vi "GetHeuristicCost.vi"(8 "error in (no error)":errorcluster, 10 "Goal NodeReference":refnum<data-value>, 11 "AbstractAstarNode in":refnum<class "NI_Robotics_AbstractAstarNode.lvclass">) -> (0 "error out":errorcluster, 2 "hueristic cost":dbl, 3 "AbstractAstarNode out":refnum<class "NI_Robotics_AbstractAstarNode.lvclass">)   [LabVIEW 2017, in "NI_Robotics_AbstractAstarNode.lvclass"]
uses:
  <vilib>/robotics/Navigation/shared/MapNode/AbstractAstarNode/NI_Robotics_AbstractAstarNode.lvclass
  <vilib>/robotics/Navigation/shared/MapNode/AbstractMapNode/NI_Robotics_AbstractMapNode.lvclass
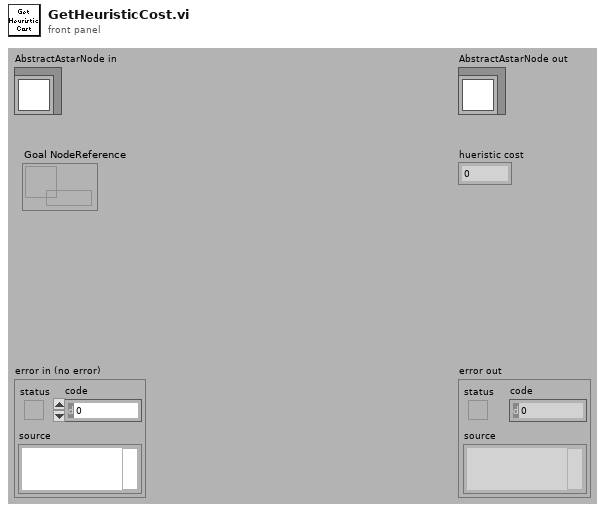
[diagram p1: front panel]
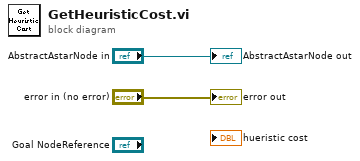
[diagram p0: block diagram]
diagram:
  "error out" <- "error in (no error)"
  "AbstractAstarNode out" <- "AbstractAstarNode in"
